vi "Write Pre-Addressed Publisher Messages.vi"(8 "Pre-Addressed Unlock Publication Msg":refnum<class "Unlock Publication Msg.lvclass">, 9 "Pre-Addressed Lock Publication Msg":refnum<class "Lock Publication Msg.lvclass">, 10 "Pre-Addressed Publish Msg":refnum<class "Publish Msg.lvclass">, 11 "IModel in":refnum<class "IModel.lvclass">) -> (3 "IModel out":refnum<class "IModel.lvclass">)   [LabVIEW 2020, in "IModel.lvlib" / "IModel.lvclass"]
doc: "<License>\nCopyright © 2017 Composed Systems, LLC | All rights reserved\nwww.composed.io\n\nAuthor: Ethan Stern <ethan.stern@composed.io>\n\nThis software is provided \"AS IS\" WITHOUT WARRANTIES, either express or implied, AND IS FOR EDUCATIONAL PURPOSES ONLY.\n</License>"
uses:
  <vilib>/gpm_packages/@cs/mva-core/Source/IModel/IModel/IModel.lvclass
  <vilib>/gpm_packages/@cs/mva-core/Source/IMediator/IMediator Messages/Publish Msg/Publish Msg.lvclass
  <vilib>/gpm_packages/@cs/mva-core/Source/IMediator/IMediator Messages/Lock Publication Msg/Lock Publication Msg.lvclass
  <vilib>/gpm_packages/@cs/mva-core/Source/IMediator/IMediator Messages/Unlock Publication Msg/Unlock Publication Msg.lvclass
  <vilib>/gpm_packages/@cs/mva-core/Source/IModel/IModel/IModel.lvclass/IModel.ctl
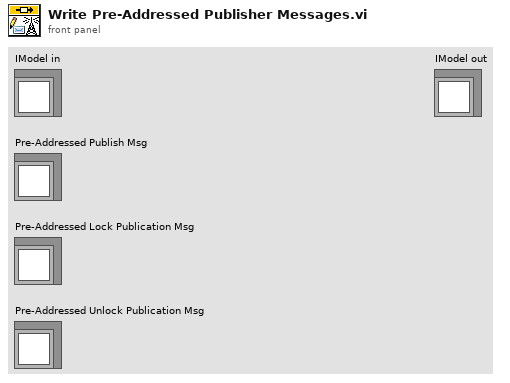
[diagram p1: front panel]
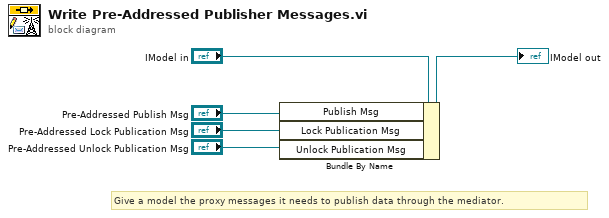
[diagram p0: block diagram]
diagram:
  # "Give a model the proxy messages it needs to publish data through the mediator."
  n1 = Bundle By Name(cluster="IModel in", "Publish Msg"="Pre-Addressed Publish Msg", "Lock Publication Msg"="Pre-Addressed Lock Publication Msg", "Unlock Publication Msg"="Pre-Addressed Unlock Publication Msg") -> (→"IModel out":refnum<class "IModel.lvclass">)
